vi "Run.vi"(8 "Column":i32, 9 "Row":i32, 10 "Maze (0: Empty, -1: Enemy. 1: Teammate)":i32[](array[numeric]), 11 "Runner in":refnum<class "Sentinel.lvclass">) -> (0 "Replicated":refnum<class "Square.lvclass">, 1 "Direction":T1, 2 "Action":T2, 3 "Runner out":refnum<class "Sentinel.lvclass">)   [LabVIEW 2015, in "Sentinel.lvclass"]
uses:
  Sentinel.lvclass
  Type Defs/Action Enum.ctl
  Type Defs/Direction Enum.ctl
  Square/Square.lvclass
  Carl/Formics/Attack Options.ctl
  Sentinel.lvclass/Sentinel.ctl
  Carl/Common/Reverse Direction.vi
  SubVIs/Read-Only Globals.vi
  Type Defs/SB Type Defs.lvlib
  Carl/Common/Common.lvlib
  Carl/Formics/Formics.lvclass
panel:
  # "NW\nN\nNE\nE\nSE\nS\nSW\nW"
  # "NOTICE - YOU MUST NOT REMOVE THIS NOTICE. PER THE FOLLOWING LICENSE, YOU MAY REPRODUCE THIS SOFTWARE PROVIDED YOU FOLLOW THE TERMS\nOF THE LICENSE.\n\n---BEGIN BSD LICENSE (http://opensource.org/licenses/BSD-2-Clause)---\nCopyright (c) 2015, Endigit, Inc. <robert@endigit.com>\nAll rights reserved.\n\nRedistribution and use in source and binary forms, with or without modification, are permitted provided that the following conditions are met:\n\n1. Redistributions of source code must retain the above copyright notice, this list of conditions and the following disclaimer.\n\n2. Redistributions in binary form must reproduce the above copyright notice, this list of conditions and the following disclaimer in the documentation and/or other \nmaterials provided with the distribution.\n\nTHIS SOFTWARE IS PROVIDED BY THE COPYRIGHT HOLDERS AND CONTRIBUTORS \"AS IS\" AND ANY EXPRESS OR IMPLIED WARRANTIES, INCLUDING, BUT NOT \nLIMITED TO, THE IMPLIED WARRANTIES OF MERCHANTABILITY AND FITNESS FOR A PARTICULAR PURPOSE ARE DISCLAIMED. IN NO EVENT SHALL THE COPYRIGHT \nHOLDER OR CONTRIBUTORS BE LIABLE FOR ANY DIRECT, INDIRECT, INCIDENTAL, SPECIAL, EXEMPLARY, OR CONSEQUENTIAL DAMAGES (INCLUDING, BUT NOT \nLIMITED TO, PROCUREMENT OF SUBSTITUTE GOODS OR SERVICES; LOSS OF USE, DATA, OR PROFITS; OR BUSINESS INTERRUPTION) HOWEVER CAUSED AND ON \nANY THEORY OF LIABILITY, WHETHER IN CONTRACT, STRICT LIABILITY, OR TORT (INCLUDING NEGLIGENCE OR OTHERWISE) ARISING IN ANY WAY OUT OF THE USE \nOF THIS SOFTWARE, EVEN IF ADVISED OF THE POSSIBILITY OF SUCH DAMAGE.\n---END BSD LICENSE---"
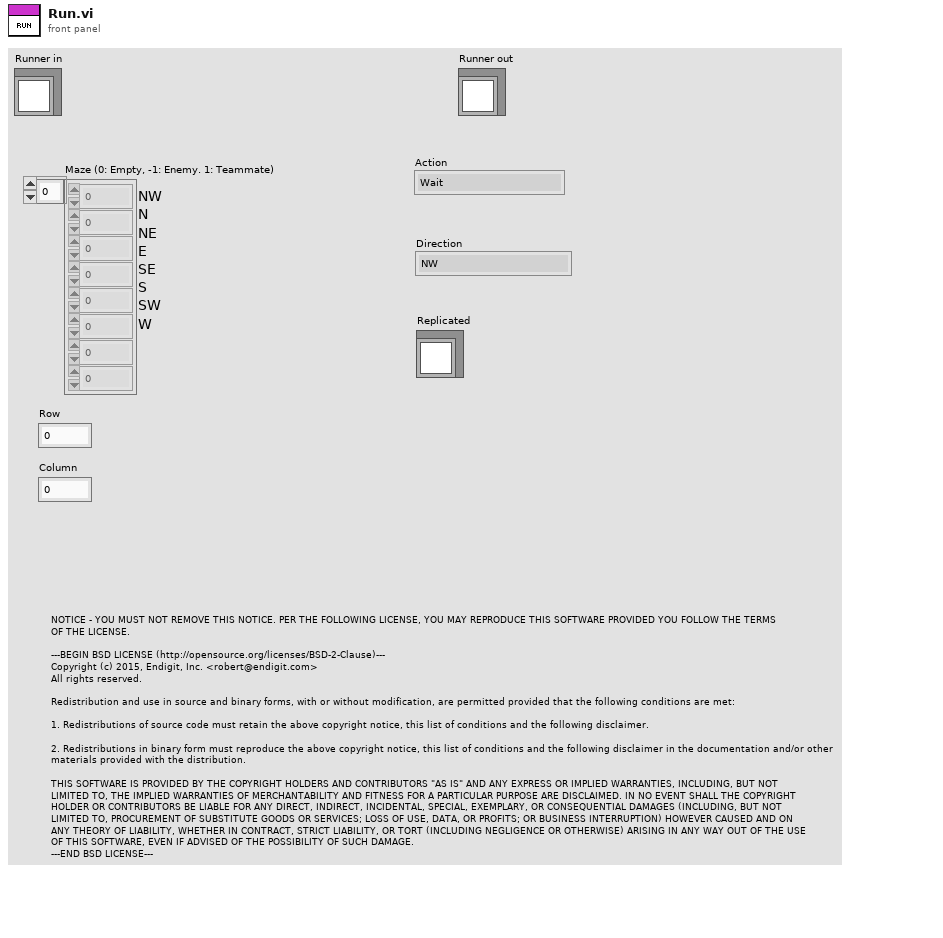
[diagram p1: front panel]
types:
  T1 = typedef "SB Type Defs.lvlib/Direction Enum.ctl" = enum16{"NW", "N", "NE", "E", "SE", "S", "SW", "W"}
  T2 = typedef "SB Type Defs.lvlib/Action Enum.ctl" = enum16{"Wait", "Move", "Attack", "Replicate"}
  T3 = typedef "Formics.lvclass/Attack Options.ctl" = enum16{"Attack", "Run", "Distract"}
  T4 = enum16{"Replicator", "Replicatee", "Eastwards", "Westwards"}
  T5 = enum16{"Replication", "Northwards", "Southwards"}
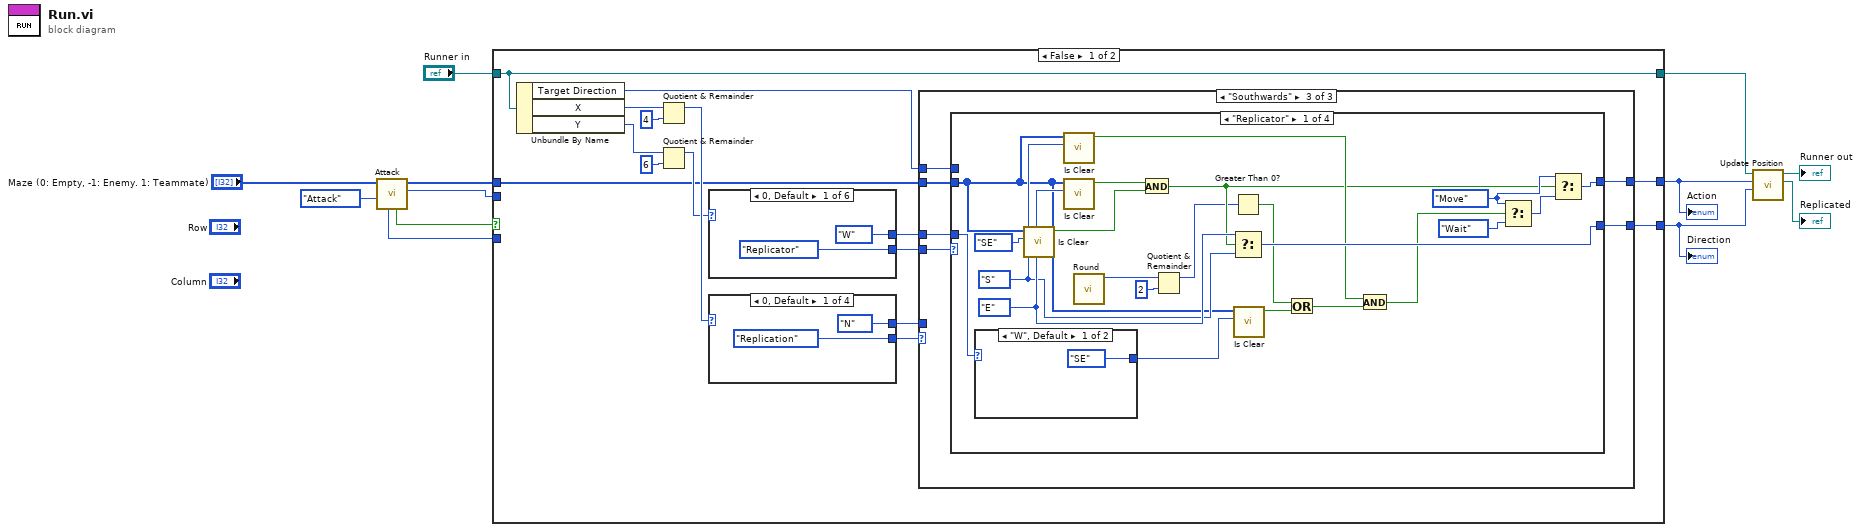
[diagram p0: block diagram]
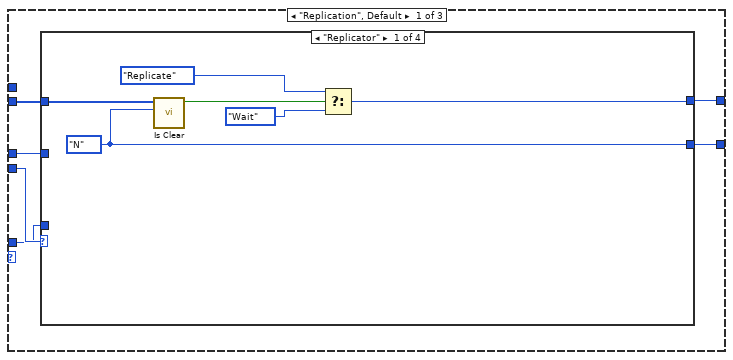
[diagram p2: hidden frame]
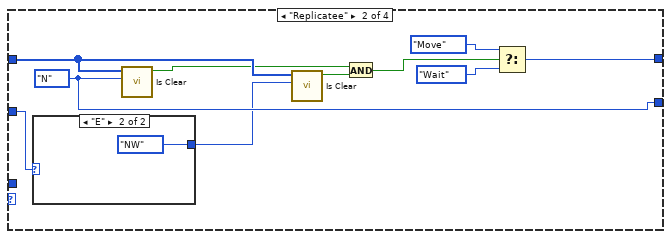
[diagram p3: hidden frame]
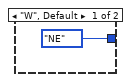
[diagram p4: hidden frame]
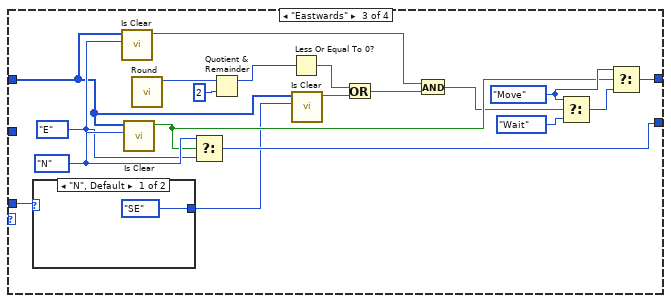
[diagram p5: hidden frame]
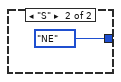
[diagram p6: hidden frame]
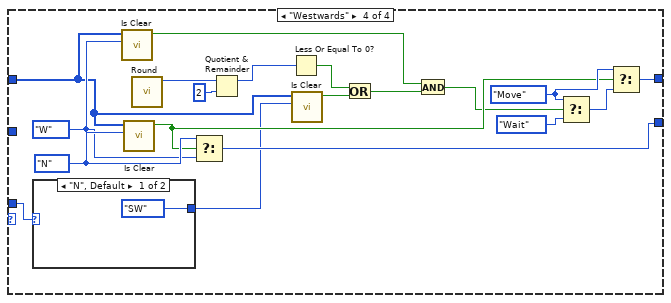
[diagram p7: hidden frame]
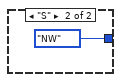
[diagram p8: hidden frame]
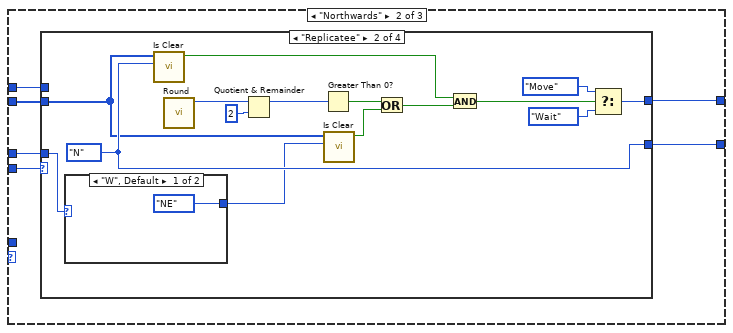
[diagram p9: hidden frame]
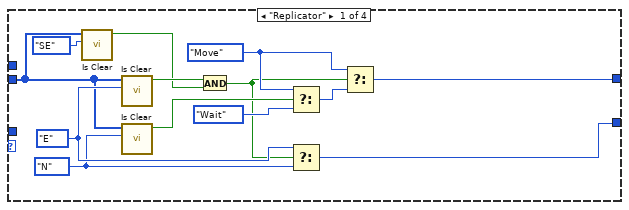
[diagram p10: hidden frame]
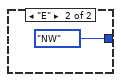
[diagram p11: hidden frame]
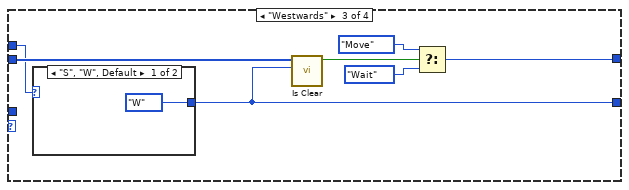
[diagram p12: hidden frame]
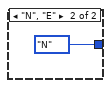
[diagram p13: hidden frame]
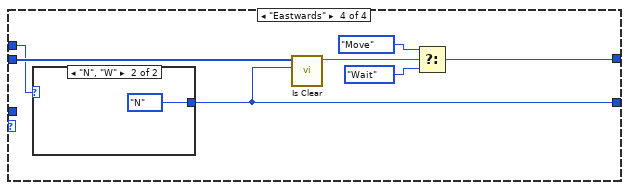
[diagram p14: hidden frame]
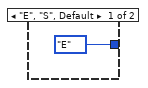
[diagram p15: hidden frame]
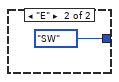
[diagram p16: hidden frame]
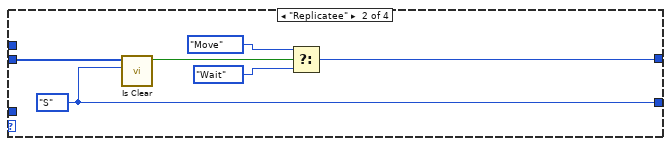
[diagram p17: hidden frame]
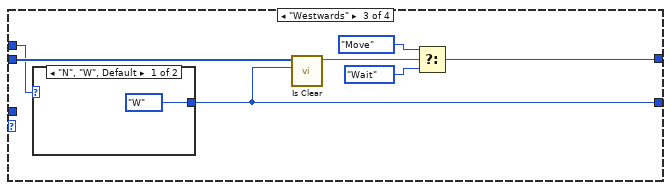
[diagram p18: hidden frame]
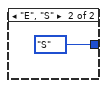
[diagram p19: hidden frame]
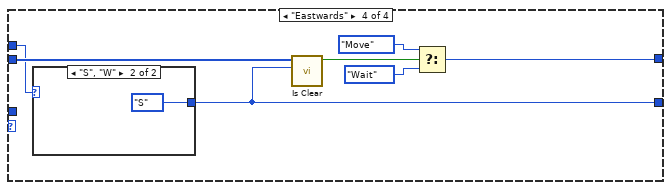
[diagram p20: hidden frame]
diagram:
  n1 = call "Attack.vi"("Attack?"=Attack_Options."Attack", "Maze (0: Empty, -1: Enemy. >0: Teammate"="Maze (0: Empty, -1: Enemy. 1: Teammate)") -> ("Action"=w11:T2, "Maze (0: Empty, -1: Enemy. >0: Teammate 2"=w8:i32[], "Enemy Found?"=w12:bool, "Enemy Direction"=w10:i32)  [unwired: 4 in, 2 out]
  n2 = case shown="False" w12 {
    tunnel: "Runner in" -> [w19 w222]
    tunnel: w11 -> [_ w224]
    tunnel: [w18 w224] -> w2
    tunnel: w10 -> [_ w223]
    tunnel: [w17 w223] -> w3
    tunnel: [w19 w222] -> w6
    tunnel: w8 -> [w16 _]
    frame False {
      n3 = Unbundle By Name(w19) -> ("Target Direction"=w14:T1, "X"=w27:i16, "Y"=w23:i16)
      n4 = Quotient & Remainder(x=w27, y=4) -> (x-y*floor(x/y)=w25:i32)  [unwired: 1 out]
      n5 = Quotient & Remainder(x=w23, y=6) -> (x-y*floor(x/y)=w22:i32)  [unwired: 1 out]
      n6 = case shown="0, Default" w22 {
        tunnel: [T4."Replicator" ("Rows") T4."Replicatee" ("Rows") T4."Eastwards" ("Rows") T4."Replicator" ("Rows") T4."Replicatee" ("Rows") T4."Westwards" ("Rows")] -> w20
        tunnel: [Direction_Enum."W" ("Direction") Direction_Enum."E" ("Direction") Direction_Enum."E" ("Direction") Direction_Enum."E" ("Direction") Direction_Enum."W" ("Direction") Direction_Enum."W" ("Direction")] -> w15
        frame 0, Default {
        }
        frame 1 {
        }
        frame 2 {
        }
        frame 3 {
        }
        frame 4 {
        }
        frame 5 {
        }
      }
      n7 = case shown="0, Default" w25 {
        tunnel: [Direction_Enum."N" ("Direction") Direction_Enum."N" ("Direction") Direction_Enum."S" ("Direction") Direction_Enum."S" ("Direction")] -> w13
        tunnel: [T5."Replication" ("Cols") T5."Northwards" ("Cols") T5."Replication" ("Cols") T5."Southwards" ("Cols")] -> w21
        frame 0, Default {
        }
        frame 1 {
        }
        frame 2 {
        }
        frame 3 {
        }
      }
      n8 = case shown="\"Southwards\"" w21 {
        tunnel: w20 -> [w33 w99 w153]
        tunnel: [w32 w98 w152] -> w18
        tunnel: [w31 w97 w151] -> w17
        tunnel: w16 -> [w30 w96 w150]
        tunnel: w15 -> [w29 w95 w149]
        tunnel: w14 -> [_ w94 w148]
        tunnel: w13 -> [w28 _ _]
        frame "Replication", Default {
          n9 = case shown="\"Replicator\"" w33 {
            tunnel: [w36 w46 w70 w91] -> w32
            tunnel: [w38 w49 w67 w88] -> w31
            tunnel: w30 -> [w39 w44 w53 w78]
            tunnel: w29 -> [_ w45 _ _]
            tunnel: w28 -> [_ _ w52 w73]
            frame "Replicator" {
              w38 = Direction_Enum."N" ("Direction")
              n10 = call "Is Clear.vi"("Direction"=w38, "Maze (0: Empty, -1: Enemy. >0: Teammate in"=w39) -> ("Is Clear"=w34:bool)  [unwired: 9 in]
              n11 = Select(t=Action_Enum."Replicate" ("Action"), s=w34, f=Action_Enum."Wait" ("Action")) -> (s? t:f=w36:T2)
            }
            frame "Replicatee" {
              w49 = Direction_Enum."N" ("Direction")
              n12 = case shown="\"E\"" w45 {
                tunnel: [Direction_Enum."NE" ("Direction") Direction_Enum."NW" ("Direction")] -> w43
                frame "W", Default {
                }
                frame "E" {
                }
              }
              n13 = call "Is Clear.vi"("Direction"=w49, "Maze (0: Empty, -1: Enemy. >0: Teammate in"=w44) -> ("Is Clear"=w41:bool)  [unwired: 9 in]
              n14 = call "Is Clear.vi"("Direction"=w43, "Maze (0: Empty, -1: Enemy. >0: Teammate in"=w44) -> ("Is Clear"=w42:bool)  [unwired: 9 in]
              n15 = And(x=w41, y=w42) -> (x .and. y?=w40:bool)
              n16 = Select(t=Action_Enum."Move" ("Action"), s=w40, f=Action_Enum."Wait" ("Action")) -> (s? t:f=w46:T2)
            }
            frame "Eastwards" {
              w68 = Direction_Enum."E" ("Direction")
              w65 = Action_Enum."Move" ("Action")
              w69 = Direction_Enum."N" ("Direction")
              n17 = case shown="\"N\", Default" w52 {
                tunnel: [Direction_Enum."SE" ("Direction") Direction_Enum."NE" ("Direction")] -> w58
                frame "N", Default {
                }
                frame "S" {
                }
              }
              n18 = call "Is Clear.vi"("Direction"=w68, "Maze (0: Empty, -1: Enemy. >0: Teammate in"=w53) -> ("Is Clear"=w57:bool)  [unwired: 9 in]
              n19 = call "Is Clear.vi"("Direction"=w69, "Maze (0: Empty, -1: Enemy. >0: Teammate in"=w53) -> ("Is Clear"=w63:bool)  [unwired: 9 in]
              n20 = call "Round.vi"() -> ("Round"=w62:i32)  [unwired: 11 in]
              n21 = Select(t=w69, s=w63, f=w68) -> (s? t:f=w67:T1)
              n22 = Quotient & Remainder(x=w62, y=2) -> (x-y*floor(x/y)=w60:i32)  [unwired: 1 out]
              n23 = Less Or Equal To 0?(x=w60) -> (x <= 0?=w59:bool)
              n24 = call "Is Clear.vi"("Direction"=w58, "Maze (0: Empty, -1: Enemy. >0: Teammate in"=w53) -> ("Is Clear"=w56:bool)  [unwired: 9 in]
              n25 = Or(x=w59, y=w56) -> (x .or. y?=w55:bool)
              n26 = And(x=w57, y=w55) -> (x .and. y?=w54:bool)
              n27 = Select(t=w65, s=w54, f=Action_Enum."Wait" ("Action")) -> (s? t:f=w64:T2)
              n28 = Select(t=w65, s=w63, f=w64) -> (s? t:f=w70:T2)
            }
            frame "Westwards" {
              w89 = Direction_Enum."W" ("Direction")
              w86 = Action_Enum."Move" ("Action")
              w90 = Direction_Enum."N" ("Direction")
              n29 = case shown="\"N\", Default" w73 {
                tunnel: [Direction_Enum."SW" ("Direction") Direction_Enum."NW" ("Direction")] -> w79
                frame "N", Default {
                }
                frame "S" {
                }
              }
              n30 = call "Is Clear.vi"("Direction"=w89, "Maze (0: Empty, -1: Enemy. >0: Teammate in"=w78) -> ("Is Clear"=w77:bool)  [unwired: 9 in]
              n31 = call "Is Clear.vi"("Direction"=w90, "Maze (0: Empty, -1: Enemy. >0: Teammate in"=w78) -> ("Is Clear"=w84:bool)  [unwired: 9 in]
              n32 = call "Round.vi"() -> ("Round"=w82:i32)  [unwired: 11 in]
              n33 = Select(t=w90, s=w84, f=w89) -> (s? t:f=w88:T1)
              n34 = Quotient & Remainder(x=w82, y=2) -> (x-y*floor(x/y)=w81:i32)  [unwired: 1 out]
              n35 = Less Or Equal To 0?(x=w81) -> (x <= 0?=w80:bool)
              n36 = call "Is Clear.vi"("Direction"=w79, "Maze (0: Empty, -1: Enemy. >0: Teammate in"=w78) -> ("Is Clear"=w76:bool)  [unwired: 9 in]
              n37 = Or(x=w80, y=w76) -> (x .or. y?=w75:bool)
              n38 = And(x=w77, y=w75) -> (x .and. y?=w74:bool)
              n39 = Select(t=w86, s=w74, f=Action_Enum."Wait" ("Action")) -> (s? t:f=w85:T2)
              n40 = Select(t=w86, s=w84, f=w85) -> (s? t:f=w91:T2)
            }
          }
        }
        frame "Northwards" {
          n41 = case shown="\"Replicatee\"" w99 {
            tunnel: [w107 w124 w133 w142] -> w98
            tunnel: [w108 w125 w130 w139] -> w97
            tunnel: w96 -> [w106 w123 w132 w141]
            tunnel: w95 -> [_ w121 _ _]
            tunnel: w94 -> [_ _ w131 w140]
            frame "Replicator" {
              w101 = Direction_Enum."N" ("Direction")
              w109 = Direction_Enum."E" ("Direction")
              w104 = Action_Enum."Move" ("Action")
              n42 = call "Is Clear.vi"("Direction"=Direction_Enum."SE", "Maze (0: Empty, -1: Enemy. >0: Teammate in"=w106) -> ("Is Clear"=w110:bool)  [unwired: 9 in]
              n43 = call "Is Clear.vi"("Direction"=w109, "Maze (0: Empty, -1: Enemy. >0: Teammate in"=w106) -> ("Is Clear"=w111:bool)  [unwired: 9 in]
              n44 = call "Is Clear.vi"("Direction"=w101, "Maze (0: Empty, -1: Enemy. >0: Teammate in"=w106) -> ("Is Clear"=w103:bool)  [unwired: 9 in]
              n45 = And(x=w111, y=w110) -> (x .and. y?=w100:bool)
              n46 = Select(t=w104, s=w103, f=Action_Enum."Wait" ("Action")) -> (s? t:f=w102:T2)
              n47 = Select(t=w109, s=w100, f=w101) -> (s? t:f=w108:T1)
              n48 = Select(t=w104, s=w100, f=w102) -> (s? t:f=w107:T2)
            }
            frame "Replicatee" {
              w125 = Direction_Enum."N" ("Direction")
              n49 = case shown="\"W\", Default" w121 {
                tunnel: [Direction_Enum."NE" ("Direction") Direction_Enum."NW" ("Direction")] -> w120
                frame "W", Default {
                }
                frame "E" {
                }
              }
              n50 = call "Is Clear.vi"("Direction"=w125, "Maze (0: Empty, -1: Enemy. >0: Teammate in"=w123) -> ("Is Clear"=w122:bool)  [unwired: 9 in]
              n51 = call "Round.vi"() -> ("Round"=w118:i32)  [unwired: 11 in]
              n52 = Quotient & Remainder(x=w118, y=2) -> (x-y*floor(x/y)=w115:i32)  [unwired: 1 out]
              n53 = Greater Than 0?(x=w115) -> (x > 0?=w114:bool)
              n54 = call "Is Clear.vi"("Direction"=w120, "Maze (0: Empty, -1: Enemy. >0: Teammate in"=w123) -> ("Is Clear"=w116:bool)  [unwired: 9 in]
              n55 = Or(x=w114, y=w116) -> (x .or. y?=w113:bool)
              n56 = And(x=w122, y=w113) -> (x .and. y?=w119:bool)
              n57 = Select(t=Action_Enum."Move" ("Action"), s=w119, f=Action_Enum."Wait" ("Action")) -> (s? t:f=w124:T2)
            }
            frame "Westwards" {
              n58 = case shown="\"S\", \"W\", Default" w131 {
                tunnel: [Direction_Enum."W" ("Direction") Direction_Enum."N" ("Direction")] -> w130
                frame "S", "W", Default {
                }
                frame "N", "E" {
                }
              }
              n59 = call "Is Clear.vi"("Direction"=w130, "Maze (0: Empty, -1: Enemy. >0: Teammate in"=w132) -> ("Is Clear"=w134:bool)  [unwired: 9 in]
              n60 = Select(t=Action_Enum."Move" ("Action"), s=w134, f=Action_Enum."Wait" ("Action")) -> (s? t:f=w133:T2)
            }
            frame "Eastwards" {
              n61 = case shown="\"N\", \"W\"" w140 {
                tunnel: [Direction_Enum."E" ("Direction") Direction_Enum."N" ("Direction")] -> w139
                frame "E", "S", Default {
                }
                frame "N", "W" {
                }
              }
              n62 = call "Is Clear.vi"("Direction"=w139, "Maze (0: Empty, -1: Enemy. >0: Teammate in"=w141) -> ("Is Clear"=w143:bool)  [unwired: 9 in]
              n63 = Select(t=Action_Enum."Move" ("Action"), s=w143, f=Action_Enum."Wait" ("Action")) -> (s? t:f=w142:T2)
            }
          }
        }
        frame "Southwards" {
          n64 = case shown="\"Replicator\"" w153 {
            tunnel: [w170 w180 w187 w196] -> w152
            tunnel: [w171 w181 w184 w193] -> w151
            tunnel: w150 -> [w165 w179 w186 w195]
            tunnel: w149 -> [w162 _ _ _]
            tunnel: w148 -> [_ _ w185 w194]
            frame "Replicator" {
              w166 = Direction_Enum."S" ("Direction")
              w172 = Direction_Enum."E" ("Direction")
              w168 = Action_Enum."Move" ("Action")
              n65 = case shown="\"W\", Default" w162 {
                tunnel: [Direction_Enum."SE" ("Direction") Direction_Enum."SW" ("Direction")] -> w161
                frame "W", Default {
                }
                frame "E" {
                }
              }
              n66 = call "Is Clear.vi"("Direction"=Direction_Enum."SE", "Maze (0: Empty, -1: Enemy. >0: Teammate in"=w165) -> ("Is Clear"=w173:bool)  [unwired: 9 in]
              n67 = call "Is Clear.vi"("Direction"=w166, "Maze (0: Empty, -1: Enemy. >0: Teammate in"=w165) -> ("Is Clear"=w164:bool)  [unwired: 9 in]
              n68 = call "Is Clear.vi"("Direction"=w172, "Maze (0: Empty, -1: Enemy. >0: Teammate in"=w165) -> ("Is Clear"=w174:bool)  [unwired: 9 in]
              n69 = call "Round.vi"() -> ("Round"=w156:i32)  [unwired: 11 in]
              n70 = And(x=w174, y=w173) -> (x .and. y?=w160:bool)
              n71 = Quotient & Remainder(x=w156, y=2) -> (x-y*floor(x/y)=w158:i32)  [unwired: 1 out]
              n72 = Greater Than 0?(x=w158) -> (x > 0?=w159:bool)
              n73 = Select(t=w172, s=w160, f=w166) -> (s? t:f=w171:T1)
              n74 = call "Is Clear.vi"("Direction"=w161, "Maze (0: Empty, -1: Enemy. >0: Teammate in"=w165) -> ("Is Clear"=w155:bool)  [unwired: 9 in]
              n75 = Or(x=w159, y=w155) -> (x .or. y?=w154:bool)
              n76 = And(x=w164, y=w154) -> (x .and. y?=w163:bool)
              n77 = Select(t=w168, s=w163, f=Action_Enum."Wait" ("Action")) -> (s? t:f=w167:T2)
              n78 = Select(t=w168, s=w160, f=w167) -> (s? t:f=w170:T2)
            }
            frame "Replicatee" {
              w181 = Direction_Enum."S" ("Direction")
              n79 = call "Is Clear.vi"("Direction"=w181, "Maze (0: Empty, -1: Enemy. >0: Teammate in"=w179) -> ("Is Clear"=w178:bool)  [unwired: 9 in]
              n80 = Select(t=Action_Enum."Move" ("Action"), s=w178, f=Action_Enum."Wait" ("Action")) -> (s? t:f=w180:T2)
            }
            frame "Westwards" {
              n81 = case shown="\"N\", \"W\", Default" w185 {
                tunnel: [Direction_Enum."W" ("Direction") Direction_Enum."S" ("Direction")] -> w184
                frame "N", "W", Default {
                }
                frame "E", "S" {
                }
              }
              n82 = call "Is Clear.vi"("Direction"=w184, "Maze (0: Empty, -1: Enemy. >0: Teammate in"=w186) -> ("Is Clear"=w188:bool)  [unwired: 9 in]
              n83 = Select(t=Action_Enum."Move" ("Action"), s=w188, f=Action_Enum."Wait" ("Action")) -> (s? t:f=w187:T2)
            }
            frame "Eastwards" {
              n84 = case shown="\"S\", \"W\"" w194 {
                tunnel: [Direction_Enum."E" ("Direction") Direction_Enum."S" ("Direction")] -> w193
                frame "N", "E", Default {
                }
                frame "S", "W" {
                }
              }
              n85 = call "Is Clear.vi"("Direction"=w193, "Maze (0: Empty, -1: Enemy. >0: Teammate in"=w195) -> ("Is Clear"=w197:bool)  [unwired: 9 in]
              n86 = Select(t=Action_Enum."Move" ("Action"), s=w197, f=Action_Enum."Wait" ("Action")) -> (s? t:f=w196:T2)
            }
          }
        }
      }
    }
    frame True {
    }
  }
  "Action" <- w2
  "Direction" <- w3
  n87 = call-dynamic "Update Position.vi"("Direction"=w3, "Action"=w2, "Sentinel in"=w6) -> ("Sentinel in 2"=→"Replicated":refnum<class "Sentinel.lvclass">, "Sentinel out"=→"Runner out":refnum<class "Sentinel.lvclass">)  [unwired: 6 in, 1 out]
